vi "Cleanup.vi"(8 "error in (no error)":errorcluster, 11 "SolutionBuilder in":refnum<class "SolutionBuilder.lvclass">) -> (0 "error out":errorcluster, 3 "SolutionBuilder out":refnum<class "SolutionBuilder.lvclass">)   [LabVIEW 2019, in "SolutionBuilder.lvlib" / "SolutionBuilder.lvclass"]
uses:
  SolutionBuilder.lvclass
  SolutionBuilder.lvclass/SolutionBuilder.ctl
  Private/ProjectItemMap.ctl
  ProjectItem/ProjectItem.lvclass
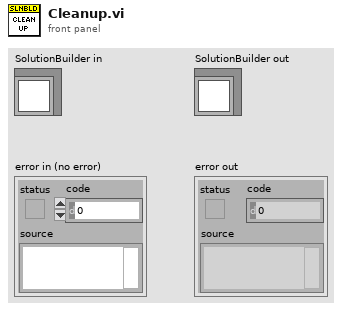
[diagram p1: front panel]
types:
  T1 = typedef "SolutionBuilder.lvlib/SolutionBuilder.lvclass/ProjectItemMap.ctl" = map{path, refnum<class "ProjectItem.lvclass">[]}
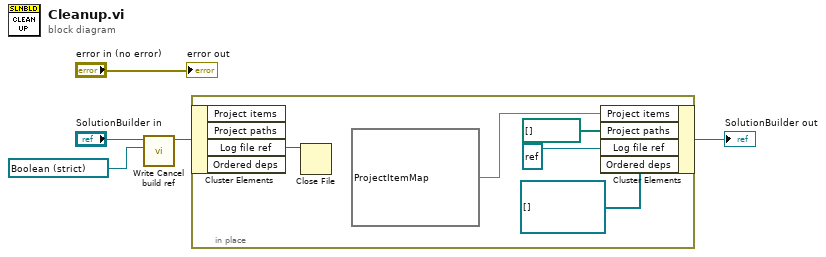
[diagram p0: block diagram]
diagram:
  n1 = call "Write Cancel build ref.vi"("Cancel build ref"=refnum<vi> refnum, "SolutionBuilder in"="SolutionBuilder in") -> ("SolutionBuilder out"=w2:refnum<class "SolutionBuilder.lvclass">)  [unwired: 9 in]
  n2 = in-place {
    n3 = in-place-cluster #1(w2) -> ("Log file ref"=w7:refnum<file>)  [unwired: 3 out]
    n4 = Close File(refnum=w7) -> ()  [unwired: 1 in, 2 out]
    n5 = in-place-cluster #1("Project items"=T1 {}, "Project paths"=path[] [], "Log file ref"=refnum<file> refnum, "Ordered deps"=refnum<class "ProjectItem.lvclass">[] []) -> (→"SolutionBuilder out":refnum<class "SolutionBuilder.lvclass">)
  }
  "error out" <- "error in (no error)"
